vi "Actor Core.vi"(8 "error in":errorcluster, 11 "Measure Object in":refnum<class "Simple Sequencer.lvclass">) -> (0 "error out":errorcluster, 3 "Actor out":refnum<class "Actor.lvclass">)   [LabVIEW 2018, in "Simple Sequencer.lvclass"]
doc: "(<B>Filename</B>: Actor Framework.lvlib:Actor.lvclass:Actor Core.vi)\n\nReceives messages to the actor, reacts to them, and initiates any error handling that may shut the actor down.\n\nDescendant classes may override this VI to append parallel tasks for the actor to complete while it handles messages. Overrides use the Call Parent Method node."
uses:
  Simple Sequencer.lvclass
  <vilib>/ActorFramework/Actor/Actor.lvclass
  Simple Sequencer Configuration.ctl
  Worker/Worker.lvclass
panel:
  in  "Configuration":T1
  out "Name":string
  # "Main sequence"
  # "Sub-sequence"
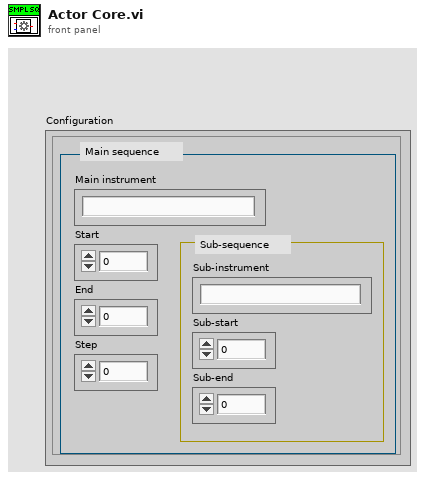
[diagram p1: front panel]
types:
  T1 = typedef "Simple Sequencer Configuration.ctl" = cluster{"Main instrument":string, "Sub-instrument":string, "Start":dbl, "End":dbl, "Step":dbl, "Sub-start":dbl, "Sub-end":dbl}
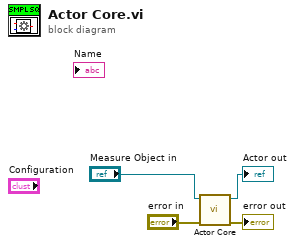
[diagram p0: block diagram]
diagram:
  n1 = call-parent "Actor Core.vi"("error in"="error in", "Measure Object in"="Measure Object in") -> ("error out"=→"error out":errorcluster, "Actor out"=→"Actor out":refnum<class "Actor.lvclass">)  [unwired: 8 in]
